vi "Main.vi"(9 "numeric":refnum<vi>, 10 "stop":refnum<vi>, 11 "get value":refnum<vi>) -> ()   [LabVIEW 2010]
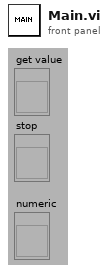
[diagram p1: front panel]
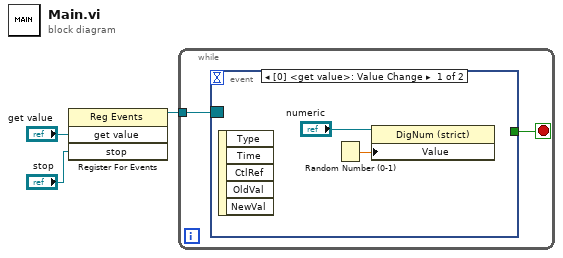
[diagram p0: block diagram]
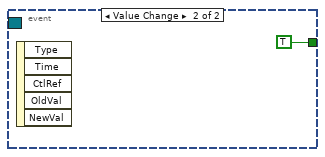
[diagram p2: hidden frame]
diagram:
  n1 = register-events("get value", "stop") -> (reference out=w3:refnum<event-registration>)  [unwired: 2 in, 1 out]
  n2 = while {
    tunnel: w3 -> [w5]
    stop <- w4 stop-if-true
    n3 = event shown="[0] <get value>: Value Change" {
      selector: w5 -> [_ _]
      dyn-events: _ -> [_ _]
      timeout: _ -> [_ _]
      tunnel: [_ TRUE] -> w4
      event Value Change {
        n4 = event-data() -> ()  [unwired: 1 in, 5 out]
        n5 = Random Number (0-1)() -> (number: 0 to 1=w6:dbl)
        n6 = property class="DigNum (strict)"(reference="numeric", "Value"=w6) -> ()  [unwired: 1 in, 2 out]
      }
      event Value Change {
        n7 = event-data() -> ()  [unwired: 1 in, 5 out]
      }
    }
  }
